vi "Initialize Core.vi"(8 "Error In":errorcluster, 11 "CS++Syslog in":refnum<class "CS++Syslog.lvclass">) -> (0 "Error Out":errorcluster, 3 "CS++Syslog out":refnum<class "CS++Syslog.lvclass">)   [LabVIEW 2016, in "CS++Syslog.lvlib" / "CS++Syslog.lvclass"]
doc: "Initialize the central message logger client."
uses:
  CS++Syslog.lvclass
  CS++Syslog.lvclass/CS++Syslog.ctl
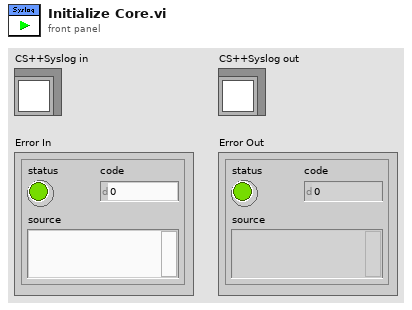
[diagram p1: front panel]
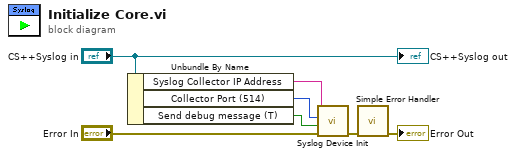
[diagram p0: block diagram]
diagram:
  n1 = Unbundle By Name("CS++Syslog in") -> ("Syslog Collector IP Address"=w3:string, "Collector Port (514)"=w4:u16, "Send debug message (T)"=w5:bool)
  n2 = call <vilib>:"Syslog Device Init.vi"("error in (no error)"="Error In", "Send debug message (T)"=w5, "Collector Port (514)"=w4, "Syslog Collector IP Address"=w3) -> ("error out"=w2:errorcluster)  [unwired: 7 in]
  n3 = call <vilib>:"Simple Error Handler.vi"("error in (no error)"=w2) -> ("error out"=→"Error Out":errorcluster)  [unwired: 4 in, 4 out]
  "CS++Syslog out" <- "CS++Syslog in"
